vi "REC_wait.vi"(4 "暂停磁铁引用":refnum<vi>, 7 "时间单位":enum16{"秒", "毫秒", "分"}(ring), 10 "停止测量引用":refnum<vi>, 11 "停留时间":dbl) -> (2 "停止？":bool)   [LabVIEW 2017]
doc: "本函数用循环等待函数的方法完成测量时在某一个位置的等待时间，这样做的好处是可以迅速终止等待。\n此外还有单位的选择。\n选择毫秒时，最快终止时间就是停留时间。\n选择秒和分时，最快终止时间为1s。"
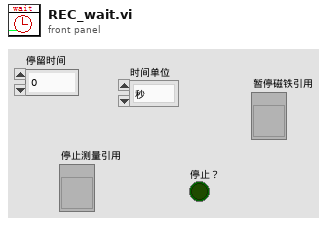
[diagram p1: front panel]
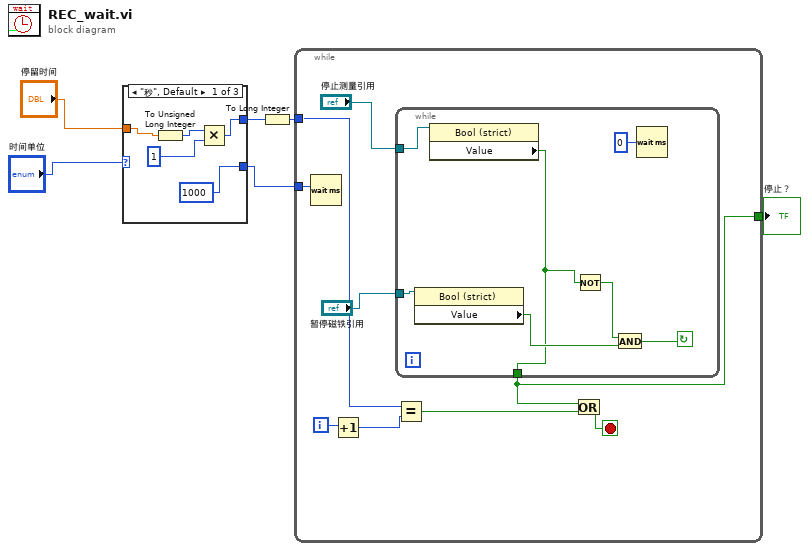
[diagram p0: block diagram]
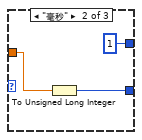
[diagram p2: hidden frame]
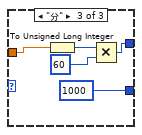
[diagram p3: hidden frame]
diagram:
  n1 = case shown="\"秒\", Default" "时间单位" {
    tunnel: [u32 1000 ("y") w12 u32 1000 ("y")] -> w3
    tunnel: "停留时间" -> [w8 w13 w17]
    tunnel: [w9 u32 1 w16] -> w4
    frame "秒", Default {
      n2 = To Unsigned Long Integer(number=w8) -> (unsigned 32bit integer=w7:u32)
      n3 = Multiply(x=w7, y=u32 1) -> (x*y=w9:u32)
    }
    frame "毫秒" {
      n4 = To Unsigned Long Integer(number=w13) -> (unsigned 32bit integer=w12:u32)
    }
    frame "分" {
      n5 = To Unsigned Long Integer(number=w17) -> (unsigned 32bit integer=w15:u32)
      n6 = Multiply(x=w15, y=u32 60) -> (x*y=w16:u32)
    }
  }
  n7 = To Long Integer(number=w4) -> (32bit integer=w2:i32)
  n8 = while {
    tunnel: w3 -> [w28]
    tunnel: w2 -> [w26]
    tunnel: [w21] -> w1
    i -> [w25]
    stop <- w23 stop-if-true
    n9 = Wait (ms)(milliseconds to wait=w28) -> ()  [unwired: 1 out]
    n10 = Increment(x=w25) -> (x+1=w27:i32)
    n11 = while {
      tunnel: "停止测量引用" -> [w35]
      tunnel: [w30] -> w21
      tunnel: "暂停磁铁引用" -> [w33]
      stop <- w31 continue-if-true
      n12 = property class="Bool (strict)"(reference=w33) -> ("Value"=w32:bool)  [unwired: 1 in, 2 out]
      n13 = property class="Bool (strict)"(reference=w35) -> ("Value"=w30:bool)  [unwired: 1 in, 2 out]
      n14 = Not(x=w30) -> (.not. x?=w29:bool)
      n15 = And(x=w29, y=w32) -> (x .and. y?=w31:bool)
      n16 = Wait (ms)(milliseconds to wait=u32 0) -> ()  [unwired: 1 out]
    }
    n17 = Equal?(x=w26, y=w27) -> (x = y?=w24:bool)
    n18 = Or(x=w21, y=w24) -> (x .or. y?=w23:bool)
  }
  "停止？" <- w1
